vi "cRIO Main.vi"() -> ()   [LabVIEW 2013]
doc: "This example runs a background service that initializes and interacts with the Tag Bus Data framework. The service is designed to run continuously so that the framework can be reinitialized with a new configuration without rebooting the target. This can save time when iterating on a configuration.\n\nThe example includes a collection of VIs for sending and receiving messages from the engine service."
uses:
  SubVIs/command commands to rtexe process.ctl
  SubVIs/engine status data.ctl
  <vilib>/NI/Module Execution Interface/Engine Runtime/Execution States.ctl
  <vilib>/NI/Module Execution Interface/Engine Runtime/Fault.ctl
  <vilib>/NI/Tag Bus Module Framework/runtime/error classification.ctl
  <vilib>/Utility/RT CPU Load.ctl
  SubVIs/queue name.ctl
  <vilib>/NI/Current Value Table/DataTypes/Double_Read.vi
  <vilib>/NI/Current Value Table/DataTypes/U32_Read.vi
  <vilib>/NI/Current Value Table/DataTypes/Boolean_Read.vi
  <vilib>/NI/Current Value Table/DataTypes/U64_Read.vi
  <vilib>/NI/Current Value Table/Type to Enum.vi
  <vilib>/NI/Current Value Table/DataTypes/Double_Type To Enum.vi
  <vilib>/NI/Current Value Table/DataTypes/U32_Type To Enum.vi
  <vilib>/NI/Current Value Table/DataTypes/Boolean_Type To Enum.vi
  <vilib>/NI/Current Value Table/DataTypes/U64_Type To Enum.vi
  <vilib>/NI/AMC/Read Termination Message.vi
  SubVIs/command to string.vi
  SubVIs/string to commands.vi
  <vilib>/NI/AMC/Create Single Message.vi
  <vilib>/NI/Current Value Table/FGVs/CVT Globals.vi
  <vilib>/NI/Current Value Table/FGVs/Tag Memory.vi
  <vilib>/NI/Current Value Table/Memory Block.vi
  <vilib>/NI/Current Value Table/DataTypes/Double_Memory Block.vi
  <vilib>/NI/Current Value Table/DataTypes/U32_Memory Block.vi
  <vilib>/NI/Current Value Table/DataTypes/Boolean_Memory Block.vi
  <vilib>/NI/Current Value Table/DataTypes/U64_Memory Block.vi
  <vilib>/NI/AMC/Globals.vi
  DCAF Execution Service.lvlib
  <vilib>/NI/AMC/AMC.lvlib
  <vilib>/NI_Real-Time Target Support.lvlib
  <vilib>/NI/Current Value Table/Current Value Table.lvlib
  <vilib>/NI/Module Execution Interface/Engine Runtime/Engine Runtime Interface.lvclass
  <vilib>/NI/Tag Bus Module Framework/runtime/TBM module execution interface.lvclass
panel:
  out "Input Time":dbl
  out "Late Count":u32
  out "Late":bool
  out "exec time":u64
  out "Loop 2 Iteration":i32
  out "Loop 1 Iteration":i32
  out "CPU loads":T1[](array[typedef]) {"ISR (%)" format="%#.2f"; "Idle (%)" format="%#.2f"; "Background (%)" format="%#.2f"; "Normal (%)" format="%#.2f"; "Above Normal (%)" format="%#.2f"; "High (%)" format="%#.2g"; "Timed Structures (%)" format="%#.2g"; "Time Critical (%)" format="%#.2g"; "Total (%)" format="%#.2g"}
  in  "target alias":string="cRIO Benchmarking"
  in  "Exit":bool
  in  "Reload":bool
  out "final error":errorcluster
  out "system error":errorcluster
  out "engine statuses":T2[](array[typedef])
  out "command error":errorcluster
  out "recent command":T6
  out "engine loaded":string
  out "load error":errorcluster
  out "invalid message":string
  in  "config. file path":path=path "/home/lvuser/Integration Testing Configuration.pcfg"
  # "status information"
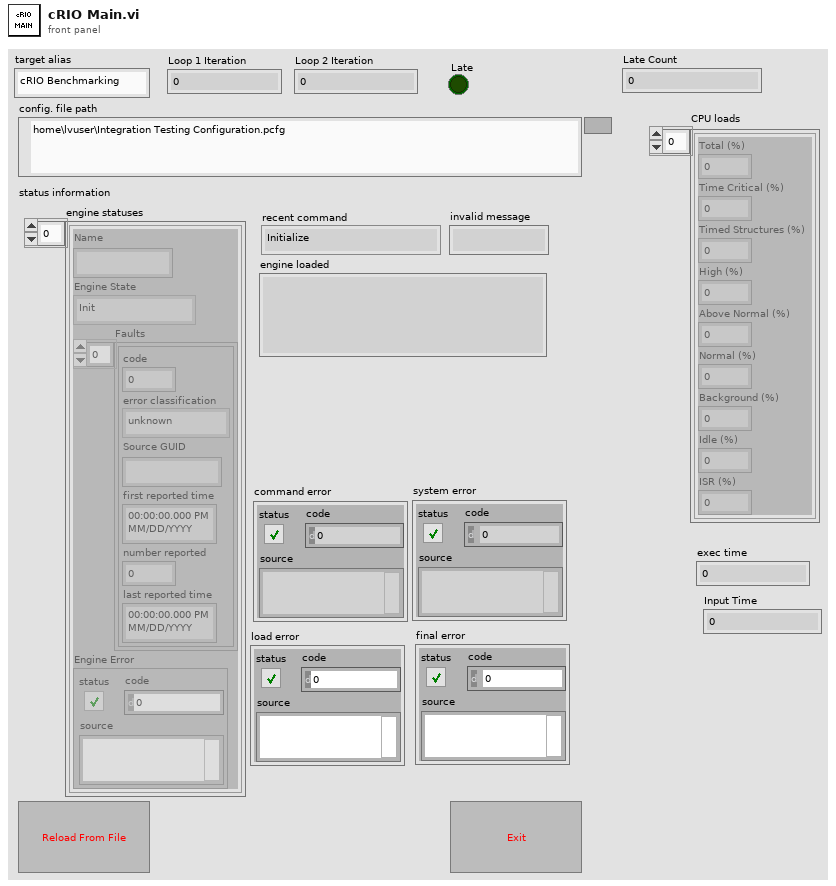
[diagram p1: front panel]
types:
  T1 = typedef "NI_Real-Time Target Support.lvlib/RT CPU Load.ctl" = cluster{"Total (%)":dbl, "Time Critical (%)":dbl, "Timed Structures (%)":dbl, "High (%)":dbl, "Above Normal (%)":dbl, "Normal (%)":dbl, "Background (%)":dbl, "Idle (%)":dbl, "ISR (%)":dbl}
  T2 = typedef "DCAF Execution Service.lvlib/engine status data.ctl" = cluster{"Name":string, "Engine State":T3, "Faults":T4[], "Engine Error":errorcluster}
  T3 = typedef "Engine Runtime Interface.lvclass/Execution States.ctl" = enum16{"Init", "Pre-Operational", "Safe-Operational", "Operational", "Stopped"}
  T4 = typedef "Engine Runtime Interface.lvclass/Fault.ctl" = cluster{"code":i32, "error classification":T5, "Source GUID":string, "first reported time":timestamp, "number reported":u32, "last reported time":timestamp}
  T5 = typedef "TBM module execution interface.lvclass/error classification.ctl" = enum16{"unknown", "none", "trivial", "recoverable", "critical"}
  T6 = typedef "DCAF Execution Service.lvlib/command commands to rtexe process.ctl" = enum16{"Initialize", "Add Search Paths", "Load from File", "Unload File", "Open All Engines", "Open Single Engine", "Initialize All Engines", "Initialize Single Engine", "Start All", "Start Single", "Pause All", "Pause Single", "Stop All", "Stop Single", "Close All", "Close Single", "Set Safe State All", "Set Safe State Single", "Get Status", "Exit", "Error", "Load Bitfile", "Unload Bitfile", "Clear Faults Single", "Clear Faults All"}
  T7 = typedef "DCAF Execution Service.lvlib/queue name.ctl" = enum16{"TOrtmainexec", "FROMrtmainexec"}
  T8 = typedef "AMC.lvlib/Message Queue.ctl" = refnum<queue>
  T9 = typedef "DCAF Execution Service.lvlib/common reponses to network process.ctl" = enum16{"System Error", "Load Report", "Action Response", "Engine Status"}
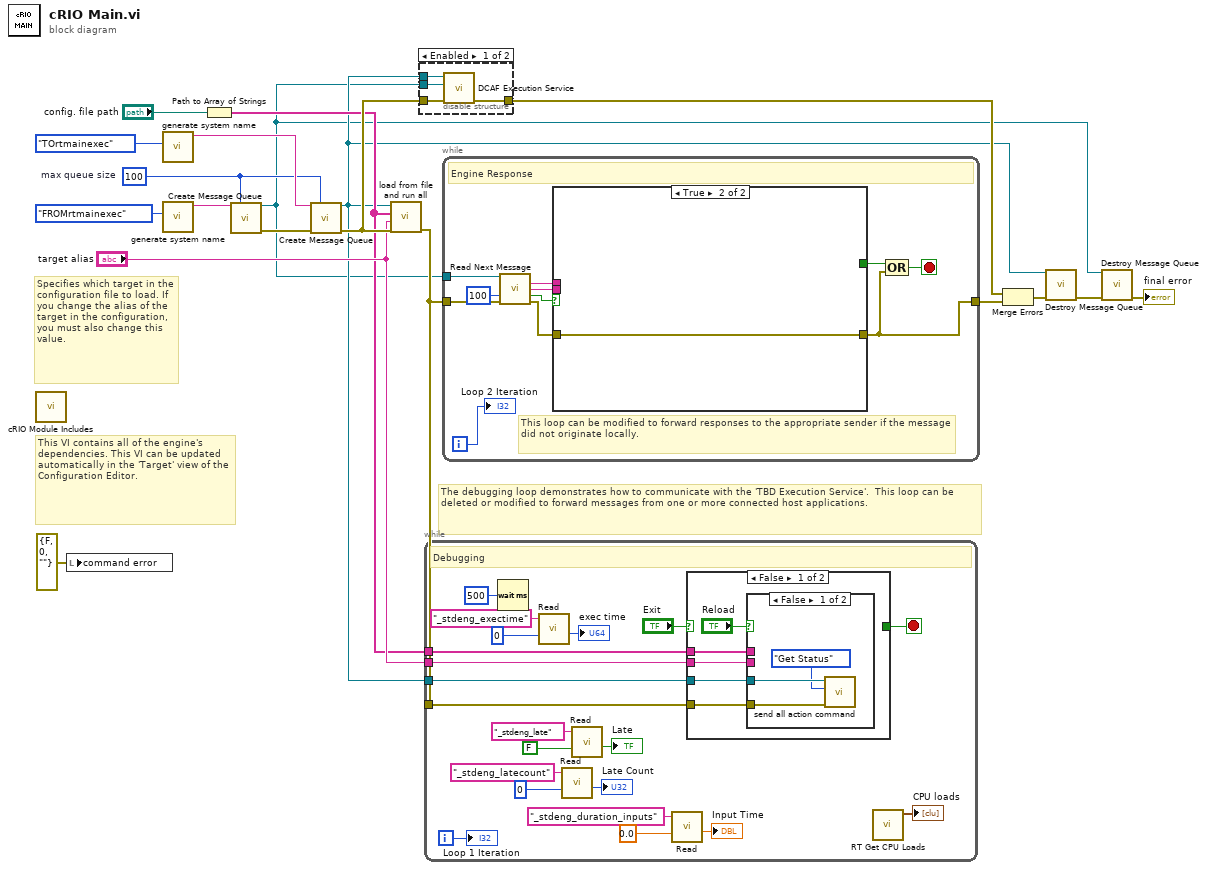
[diagram p0: block diagram]
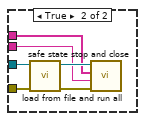
[diagram p3: hidden frame]
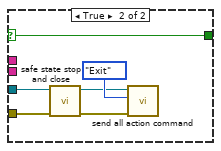
[diagram p4: hidden frame]
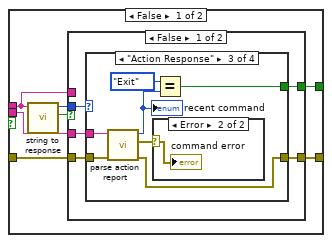
[diagram p5: hidden frame]
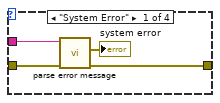
[diagram p6: hidden frame]
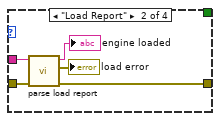
[diagram p7: hidden frame]
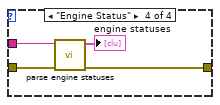
[diagram p9: hidden frame]
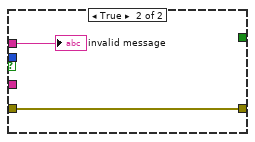
[diagram p10: hidden frame]
diagram:
  w13 = 100  # max queue size
  # "This VI contains all of the engine's dependencies. This VI can be updated automatically in the 'Target' view of the Configuration Editor."
  # "Specifies which target in the configuration file to load. If you change the alias of the target in the configuration, you must also change this value."
  # "The debugging loop demonstrates how to communicate with the 'TBD Execution Service'.  This loop can be deleted or modified to forward messages from one or more connected host applications."
  n1 = call "cRIO Module Includes.vi"() -> ()  [unwired: 12 in]
  n2 = local write "command error"(errorcluster {"status"=FALSE, "code"=0, "source"=""} ("command error")) -> ()
  n3 = call "generate system name.vi"("queue type"=queue_name."TOrtmainexec" ("queue")) -> ("queue name"=w17:string)  [unwired: 10 in]
  n4 = call "generate system name.vi"("queue type"=queue_name."FROMrtmainexec" ("queue")) -> ("queue name"=w19:string)  [unwired: 10 in]
  n5 = Path to Array of Strings(0:"config. file path") -> (2:w9:string[])  [unwired: 1 out]
  n6 = call <vilib>:"Create Message Queue.vi"("message queue name"=w19, "max queue size (-1, unlimited)"=w13) -> ("message queue out"=w2:T8, "error out"=w18:errorcluster)  [unwired: 12 in]
  n7 = call <vilib>:"Create Message Queue.vi"("message queue name"=w17, "max queue size (-1, unlimited)"=w13, "error in"=w18) -> ("message queue out"=w3:T8, "error out"=w12:errorcluster)  [unwired: 11 in]
  n8 = call "load from file and run all.vi"("error in"=w12, "target alias"="target alias", "tokenized path"=w9, "message queue in"=w3) -> ("error out"=w11:errorcluster)  [unwired: 6 in, 1 out]
  n9 = disable-structure shown="Enabled" {
    disable-tunnel: w12 -> [w23 _]
    disable-tunnel: [w22 _] -> w7
    disable-tunnel: w3 -> [w21 _]
    disable-tunnel: w2 -> [w20 _]
    frame Enabled {
      n10 = call "DCAF Execution Service.vi"("error in"=w23, "response queue"=w20, "command queue"=w21) -> ("error out"=w22:errorcluster)  [unwired: 8 in]
    }
    frame Disabled {
    }
  }
  n11 = while {
    tunnel: w11 -> [w42]
    tunnel: w3 -> [w43]
    tunnel: w9 -> [w41]
    tunnel: "target alias" -> [w40]
    i -> [w36]
    stop <- w39 stop-if-true
    # "Debugging"
    n12 = Wait (ms)(milliseconds to wait=u32 500) -> ()  [unwired: 1 out]
    n13 = call-poly <vilib>:"Read.vi"("Default"=u64 0, "Tag Name"="_stdeng_exectime") -> ("Value"=→"exec time":u64)  [unwired: 8 in, 1 out]
    n14 = call-poly <vilib>:"Read.vi"("Default"=u32 0, "Tag Name"="_stdeng_latecount") -> ("Value"=→"Late Count":u32)  [unwired: 8 in, 1 out]
    n15 = call-poly <vilib>:"Read.vi"("Default"=FALSE, "Tag Name"="_stdeng_late") -> ("Value"=→"Late":bool)  [unwired: 8 in, 1 out]
    n16 = call-poly <vilib>:"Read.vi"("Default"=0.0, "Tag Name"="_stdeng_duration_inputs") -> ("Value"=→"Input Time":dbl)  [unwired: 8 in, 1 out]
    n17 = case shown="False" "Exit" {
      selector: "Exit" -> [_ w62]
      tunnel: w43 -> [w48 w64]
      tunnel: w42 -> [w47 w63]
      tunnel: w41 -> [w46 _]
      tunnel: w40 -> [w45 _]
      tunnel: [_ w62] -> w39
      frame False {
        n18 = case shown="False" "Reload" {
          tunnel: w48 -> [w52 w58]
          tunnel: w47 -> [w51 w57]
          tunnel: w46 -> [_ w54]
          tunnel: w45 -> [_ w53]
          frame False {
            n19 = call "send all action command.vi"("error in"=w51, "commands"=command_commands_to_rtexe_process."Get Status", "message queue in"=w52) -> ()  [unwired: 7 in, 2 out]
          }
          frame True {
            n20 = call "safe state stop and close.vi"("error in"=w57, "message queue in"=w58) -> ("error out"=w55:errorcluster, "message queue out"=w56:T8)  [unwired: 8 in]
            n21 = call "load from file and run all.vi"("error in"=w55, "target alias"=w53, "tokenized path"=w54, "message queue in"=w56) -> ()  [unwired: 6 in, 2 out]
          }
        }
      }
      frame True {
        n22 = call "safe state stop and close.vi"("error in"=w63, "message queue in"=w64) -> ("error out"=w59:errorcluster, "message queue out"=w60:T8)  [unwired: 8 in]
        n23 = call "send all action command.vi"("error in"=w59, "commands"=command_commands_to_rtexe_process."Exit", "message queue in"=w60) -> ()  [unwired: 7 in, 2 out]
      }
    }
    n24 = call <vilib>:"RT Get CPU Loads.vi"() -> ("CPU loads"=→"CPU loads":T1[])  [unwired: 10 in, 1 out]
    "Loop 1 Iteration" <- w36
  }
  n25 = while {
    tunnel: w2 -> [w74]
    tunnel: w11 -> [w71]
    tunnel: [w66] -> w8
    i -> [w65]
    stop <- w68 stop-if-true
    # "This loop can be modified to forward responses to the appropriate sender if the message did not originate locally."
    # "Engine Response"
    n26 = call <vilib>:"Read Next Message.vi"("message queue in"=w74, "timeout (1 ms)"=100, "error in"=w71) -> ("message name"=w73:string, "message value"=w67:string, "timed out?"=w70:bool, "error out"=w72:errorcluster)  [unwired: 5 in, 4 out]
    n27 = case shown="True" w70 {
      tunnel: w73 -> [w76 _]
      tunnel: [w81 _] -> w69
      tunnel: w72 -> [w79 w111]
      tunnel: [w78 w111] -> w66
      tunnel: w67 -> [w77 _]
      frame False {
        n28 = call "string to response.vi"("command string"=w76) -> ("invalid"=w82:bool, "responses"=w80:T9)  [unwired: 9 in]
        n29 = case shown="False" w82 {
          tunnel: w77 -> [w86 _]
          tunnel: [w83 _] -> w81
          tunnel: w80 -> [w87 _]
          tunnel: w79 -> [w85 w110]
          tunnel: [w84 w110] -> w78
          tunnel: w76 -> [_ w109]
          frame False {
            n30 = case shown="\"Action Response\"" w87 {
              tunnel: w86 -> [w91 w96 w103 w108]
              tunnel: w85 -> [w90 w95 w102 w107]
              tunnel: [w88 w92 w97 w106] -> w84
              tunnel: [_ _ w99 _] -> w83
              frame "System Error" {
                n31 = call "parse error message.vi"("error in"=w90, "message data"=w91) -> ("error out"=w88:errorcluster, "system error"=→"system error":errorcluster)  [unwired: 8 in]
              }
              frame "Load Report" {
                n32 = call "parse load report.vi"("error in"=w95, "message data"=w96) -> ("error out"=w92:errorcluster, "load error"=→"load error":errorcluster, "engine loaded"=→"engine loaded":string)  [unwired: 7 in]
              }
              frame "Action Response" {
                n33 = call "parse action report.vi"("error in"=w102, "message data"=w103) -> ("error out"=w97:errorcluster, "command error"=w98:errorcluster, "commands"=w101:T6)  [unwired: 7 in]
                "recent command" <- w101
                n34 = case shown="Error" w98 {
                  selector: w98 -> [_ w104]
                  frame No Error {
                  }
                  frame Error {
                    "command error" <- w104
                  }
                }
                n35 = Equal?(x=command_commands_to_rtexe_process."Exit", y=w101) -> (x = y?=w99:bool)
              }
              frame "Engine Status" {
                n36 = call "parse engine statuses.vi"("error in"=w107, "message data"=w108) -> ("error out"=w106:errorcluster, "engine statuses"=→"engine statuses":T2[])  [unwired: 8 in]
              }
            }
          }
          frame True {
            "invalid message" <- w109
          }
        }
      }
      frame True {
      }
    }
    n37 = Compound Arithmetic op=OR(w69, w66) -> (w68:bool)
    "Loop 2 Iteration" <- w65
  }
  n38 = Merge Errors(w7, w8) -> (w4:errorcluster)
  n39 = call <vilib>:"Destroy Message Queue.vi"("message queue in"=w3, "error in"=w4) -> ("error out"=w6:errorcluster)  [unwired: 11 in, 2 out]
  n40 = call <vilib>:"Destroy Message Queue.vi"("message queue in"=w2, "error in"=w6) -> ("error out"=→"final error":errorcluster)  [unwired: 11 in, 2 out]
